vi "Mode_1.vi"(8 "error in (no error)":errorcluster, 11 "SetupInfo_IN":T1={"ConfigParameters_Analog"={"JAI camera fps"=240.0, "Bi-Lateral Galvo xy scan range (V)"=0.7, "Bi-Lateral Galvo xy scan frequency (Hz)"=500, "AOM Blind percent (%)"=0.1, "AOM start blind percent (%) "=70.0, "ROI threshold"=1.0, "AO Sampling rate"=1000000.0}, "ConfigParameters_Digital"={"Steps per volume"=25.0, "Time per volume (s)"=0.4, "OG start layer"=15.0, "Objective Lin Rising Vel (micron/ms）"=1.0, "Image depth (micron)"=200.0, "OG latency (s)"=10.0, "OG repitation"=3.0, "OG end layer"=17.0, "Shock1 duration (s)"=0.001, "Shock2 duration (s)"=0.001, "Shock3 duration (s)"=0.01, "Shock4 duration (s)"=0.01, "Shock5 duration (s)"=0.1, "Shock duration_New"=[]}, "ConfigParameters_Other1"={"Frontal Galvo xy scan range (V)"=0.14, "Frontal Galvo xy scan frequency (Hz)"=500, "PFI 0 digital clock frequency"=500000.0, "Window size for layer index"=0.5, "sCMOS fps"=95.0}, "ConfigParameters_Others2"={"#Trials baseline"=6, "#Trials test"=6, "Time before acq. (s)"=360.0, "Time before test (s)"=600.0, "#Blocks acquisition"=5, "Inter-trial interval baseline (s)"=60.0, "#Trials per acquition block"=6, "Inter-block interval acquisition (s)"=360.0, "Inter-trial interval acquisition (s)"=20.0, "Flash latency (s)"=10.0, "Flash duration (s)"=3.2, "Response duration (s)"=10.0, "MaxTimeEventDetection (s)"=6, "StimType"=enum."Flash", "#MaxEvents"=6}, "ProcessParametersOut"={"stand Z vol Acquisition time (s)"=0.2631578947368421, "stand Z vol Backward time (s)"=0.13684210526315793, "Objective scan volt"=5.0, "Bi-lateral Galvo Z scan volt"=0.1800000180000018, "Frontal Galvo Z scan volt"=0.14940000509752818, "Objective step length (micron)"=8.0, "OG Z volet Linear Dec time (s)"=0.024, "OG Z vol Stim. steps time (s)"=0.031578947368421054, "OG Z vol Linear Acc time (s)"=0.112, "#Vol. of flash"=8, "#Vol. of shock"=1, "#Vol. bef flash"=25, "#Vol. aft flash"=17, "OG Z vol Linear Dec time (s)"=0.112, "OG Z vol time (s)"=0.39073684210526316, "Stack duration"=[0.001, 0.001, 0.01, 0.01, 0.1], "AOM stand. value size"=400000, "Plane indexing length"=0, "#Vol. blank"=0, "#Vol. blank before acq"=0, "#Vol. blank before test"=0, " #Inter-block interval acquisition (Ed-St Vol)"=0}, "WaveformParameters"={"stand Z vol Acquisition samp info"={"Fs"=1000000.0, "#s"=263158.0}, "stand Z vol Backward samp info"={"Fs"=1000000.0, "#s"=136842.0}, "OG Z vol Linear Acc samp info"={"Fs"=1000000.0, "#s"=112000.0}, "OG Z vol Stim. steps samp info"={"Fs"=1000000.0, "#s"=31579.0}, "OG Z volet Linear Dec samp info"={"Fs"=1000000.0, "#s"=24000.0}, "OG Z vol Linear Dec samp info"={"Fs"=1000000.0, "#s"=112000.0}, "OG Z vol samp info"={"Fs"=1000000.0, "#s"=390737.0}, "stand Z vol backforth samp info"={"Fs"=1000000.0, "#s"=400000.0}}, "AnalogWaveform"={"Bi-lateral Galvo Z stand waveform"={"t0"=timestamp(0 s since 1904-01-01), "dt"=1.0, "Y"=[]}, "Frontal Galvo Z stand waveform"={"t0"=timestamp(0 s since 1904-01-01), "dt"=1.0, "Y"=[]}, "Bi-lateral Galvo XY stand waveform"={"t0"=timestamp(0 s since 1904-01-01), "dt"=1.0, "Y"=[]}, "Frontal Galvo XY stand waveform"={"t0"=timestamp(0 s since 1904-01-01), "dt"=1.0, "Y"=[]}, "sCMOS stand waveform"={"t0"=timestamp(0 s since 1904-01-01), "dt"=1.0, "Y"=[]}, "Detection objective stand waveform"={"t0"=timestamp(0 s since 1904-01-01), "dt"=1.0, "Y"=[]}, "AOM stand waveform"={"t0"=timestamp(0 s since 1904-01-01), "dt"=1.0, "Y"=[]}, "PFI 0 clock stand waveform"={"t0"=timestamp(0 s since 1904-01-01), "dt"=1.0, "Y"=[]}, "Bi-lateral Galvo Z OG waveform"={"t0"=timestamp(0 s since 1904-01-01), "dt"=1.0, "Y"=[]}, "Bi-lateral Galvo XY OG waveform"={"t0"=timestamp(0 s since 1904-01-01), "dt"=1.0, "Y"=[]}, "Frontal Galvo Z OG waveform"={"t0"=timestamp(0 s since 1904-01-01), "dt"=1.0, "Y"=[]}, "Frontal Galvo XY OG waveform"={"t0"=timestamp(0 s since 1904-01-01), "dt"=1.0, "Y"=[]}, "sCMOS OG waveform"={"t0"=timestamp(0 s since 1904-01-01), "dt"=1.0, "Y"=[]}, "Detection objective OG waveform"={"t0"=timestamp(0 s since 1904-01-01), "dt"=1.0, "Y"=[]}, "AOM OG waveform"={"t0"=timestamp(0 s since 1904-01-01), "dt"=1.0, "Y"=[]}, "PFI 0 clock OG wavee"={"t0"=timestamp(0 s since 1904-01-01), "dt"=1.0, "Y"=[]}, "sCMOS blank waveform"={"t0"=timestamp(0 s since 1904-01-01), "dt"=1.0, "Y"=[]}, "All analog OG wave"=[], "All analog stand wave"=[], "All analog blank wave"=[], "BufferWaveform_Analog"=[], "Bi-lateral Galvo Z XY"={"t0"=timestamp(0 s since 1904-01-01), "dt"=1.0, "Y"=[]}, "Frontal Galvo Z XY"={"t0"=timestamp(0 s since 1904-01-01), "dt"=1.0, "Y"=[]}, "sCMOS Trigger XY"={"t0"=timestamp(0 s since 1904-01-01), "dt"=1.0, "Y"=[]}, "Detection objective XY"={"t0"=timestamp(0 s since 1904-01-01), "dt"=1.0, "Y"=[]}, "AOM XY"={"t0"=timestamp(0 s since 1904-01-01), "dt"=1.0, "Y"=[]}, "Analog_XY"=[]}, "DigitalWaveform"={"AllDigitalStandWave"=[], "AllDigialEvokedWave"=[], "AllDigialOGWave"=[], "AllDigitalPairWave_1"=[], "AllDigitalPairWave_2"=[], "AllDigitalPairWave_3"=[], "AllDigitalPairWave_4"=[], "AllDigitalPairWave_5"=[], "Plane Indexing"={"t0"=timestamp(0 s since 1904-01-01), "dt"=0.0, "Y"={"transitions"=[], "data"=[]}, "error"={"status"=FALSE, "code"=37421928, "source"=""}}, "Plane indexing P0.5 OG"={"t0"=timestamp(0 s since 1904-01-01), "dt"=0.0, "Y"={"transitions"=[], "data"=[]}, "error"={"status"=FALSE, "code"=37421928, "source"=""}}, "AllDigitalPairWaves"=[], "BufferWaveform_Digital"=[], "AllDigitalBlankWave"=[], "Digial_XY"=[], "Digital_XY_flash"=[], "Digial_XY DMD"=[]}, "PhysicalResource"={"PhysicalChannels_AI"="", "PhysicalChannels_AO"="", "PhysicalChannels_DO"="", "Task_AnalogOutput"="", "Task_DigitalOutput"="", "Task_AnalogInput"=""}, "ControlsRef"={"Mode_1"=refnum, "EventDetectionMode"=refnum, "Mode_2A"=refnum, "StimulationMode"=refnum, "Mode_2B"=refnum, "ErrorMeg"=refnum}, "test"=""} {"ConfigParameters_Other1"."Frontal Galvo xy scan frequency (Hz)" min=500 max=500; "ConfigParameters_Other1"."Frontal Galvo xy scan range (V)" min=0.0 max=1.5; "ConfigParameters_Analog"."AOM start blind percent (%)" min=10.0 max=90.0; "ConfigParameters_Analog"."AOM Blind percent (%)" min=0.1 max=100.0; "ConfigParameters_Analog"."Bi-Lateral Galvo xy scan frequency (Hz)" min=500 max=500; "ConfigParameters_Analog"."Bi-Lateral Galvo xy scan range (V)" min=0.0 max=1.5}) -> (0 "error out":errorcluster, 3 "SetupInfo_OUT":T1={"ConfigParameters_Analog"={"JAI camera fps"=240.0, "Bi-Lateral Galvo xy scan range (V)"=0.7, "Bi-Lateral Galvo xy scan frequency (Hz)"=500, "AOM Blind percent (%)"=0.1, "AOM start blind percent (%) "=70.0, "ROI threshold"=1.0, "AO Sampling rate"=1000000.0}, "ConfigParameters_Digital"={"Steps per volume"=25.0, "Time per volume (s)"=0.4, "OG start layer"=15.0, "Objective Lin Rising Vel (micron/ms）"=1.0, "Image depth (micron)"=200.0, "OG latency (s)"=10.0, "OG repitation"=3.0, "OG end layer"=17.0, "Shock1 duration (s)"=0.001, "Shock2 duration (s)"=0.001, "Shock3 duration (s)"=0.01, "Shock4 duration (s)"=0.01, "Shock5 duration (s)"=0.1, "Shock duration_New"=[]}, "ConfigParameters_Other1"={"Frontal Galvo xy scan range (V)"=0.14, "Frontal Galvo xy scan frequency (Hz)"=500, "PFI 0 digital clock frequency"=500000.0, "Window size for layer index"=0.5, "sCMOS fps"=95.0}, "ConfigParameters_Others2"={"#Trials baseline"=6, "#Trials test"=6, "Time before acq. (s)"=360.0, "Time before test (s)"=600.0, "#Blocks acquisition"=5, "Inter-trial interval baseline (s)"=60.0, "#Trials per acquition block"=6, "Inter-block interval acquisition (s)"=360.0, "Inter-trial interval acquisition (s)"=20.0, "Flash latency (s)"=10.0, "Flash duration (s)"=3.2, "Response duration (s)"=10.0, "MaxTimeEventDetection (s)"=6, "StimType"=enum."Flash", "#MaxEvents"=6}, "ProcessParametersOut"={"stand Z vol Acquisition time (s)"=0.2631578947368421, "stand Z vol Backward time (s)"=0.13684210526315793, "Objective scan volt"=5.0, "Bi-lateral Galvo Z scan volt"=0.1800000180000018, "Frontal Galvo Z scan volt"=0.14940000509752818, "Objective step length (micron)"=8.0, "OG Z volet Linear Dec time (s)"=0.024, "OG Z vol Stim. steps time (s)"=0.031578947368421054, "OG Z vol Linear Acc time (s)"=0.112, "#Vol. of flash"=8, "#Vol. of shock"=1, "#Vol. bef flash"=25, "#Vol. aft flash"=17, "OG Z vol Linear Dec time (s)"=0.112, "OG Z vol time (s)"=0.39073684210526316, "Stack duration"=[0.001, 0.001, 0.01, 0.01, 0.1], "AOM stand. value size"=400000, "Plane indexing length"=0, "#Vol. blank"=0, "#Vol. blank before acq"=0, "#Vol. blank before test"=0, " #Inter-block interval acquisition (Ed-St Vol)"=0}, "WaveformParameters"={"stand Z vol Acquisition samp info"={"Fs"=1000000.0, "#s"=263158.0}, "stand Z vol Backward samp info"={"Fs"=1000000.0, "#s"=136842.0}, "OG Z vol Linear Acc samp info"={"Fs"=1000000.0, "#s"=112000.0}, "OG Z vol Stim. steps samp info"={"Fs"=1000000.0, "#s"=31579.0}, "OG Z volet Linear Dec samp info"={"Fs"=1000000.0, "#s"=24000.0}, "OG Z vol Linear Dec samp info"={"Fs"=1000000.0, "#s"=112000.0}, "OG Z vol samp info"={"Fs"=1000000.0, "#s"=390737.0}, "stand Z vol backforth samp info"={"Fs"=1000000.0, "#s"=400000.0}}, "AnalogWaveform"={"Bi-lateral Galvo Z stand waveform"={"t0"=timestamp(0 s since 1904-01-01), "dt"=1.0, "Y"=[]}, "Frontal Galvo Z stand waveform"={"t0"=timestamp(0 s since 1904-01-01), "dt"=1.0, "Y"=[]}, "Bi-lateral Galvo XY stand waveform"={"t0"=timestamp(0 s since 1904-01-01), "dt"=1.0, "Y"=[]}, "Frontal Galvo XY stand waveform"={"t0"=timestamp(0 s since 1904-01-01), "dt"=1.0, "Y"=[]}, "sCMOS stand waveform"={"t0"=timestamp(0 s since 1904-01-01), "dt"=1.0, "Y"=[]}, "Detection objective stand waveform"={"t0"=timestamp(0 s since 1904-01-01), "dt"=1.0, "Y"=[]}, "AOM stand waveform"={"t0"=timestamp(0 s since 1904-01-01), "dt"=1.0, "Y"=[]}, "PFI 0 clock stand waveform"={"t0"=timestamp(0 s since 1904-01-01), "dt"=1.0, "Y"=[]}, "Bi-lateral Galvo Z OG waveform"={"t0"=timestamp(0 s since 1904-01-01), "dt"=1.0, "Y"=[]}, "Bi-lateral Galvo XY OG waveform"={"t0"=timestamp(0 s since 1904-01-01), "dt"=1.0, "Y"=[]}, "Frontal Galvo Z OG waveform"={"t0"=timestamp(0 s since 1904-01-01), "dt"=1.0, "Y"=[]}, "Frontal Galvo XY OG waveform"={"t0"=timestamp(0 s since 1904-01-01), "dt"=1.0, "Y"=[]}, "sCMOS OG waveform"={"t0"=timestamp(0 s since 1904-01-01), "dt"=1.0, "Y"=[]}, "Detection objective OG waveform"={"t0"=timestamp(0 s since 1904-01-01), "dt"=1.0, "Y"=[]}, "AOM OG waveform"={"t0"=timestamp(0 s since 1904-01-01), "dt"=1.0, "Y"=[]}, "PFI 0 clock OG wavee"={"t0"=timestamp(0 s since 1904-01-01), "dt"=1.0, "Y"=[]}, "sCMOS blank waveform"={"t0"=timestamp(0 s since 1904-01-01), "dt"=1.0, "Y"=[]}, "All analog OG wave"=[], "All analog stand wave"=[], "All analog blank wave"=[], "BufferWaveform_Analog"=[], "Bi-lateral Galvo Z XY"={"t0"=timestamp(0 s since 1904-01-01), "dt"=1.0, "Y"=[]}, "Frontal Galvo Z XY"={"t0"=timestamp(0 s since 1904-01-01), "dt"=1.0, "Y"=[]}, "sCMOS Trigger XY"={"t0"=timestamp(0 s since 1904-01-01), "dt"=1.0, "Y"=[]}, "Detection objective XY"={"t0"=timestamp(0 s since 1904-01-01), "dt"=1.0, "Y"=[]}, "AOM XY"={"t0"=timestamp(0 s since 1904-01-01), "dt"=1.0, "Y"=[]}, "Analog_XY"=[]}, "DigitalWaveform"={"AllDigitalStandWave"=[], "AllDigialEvokedWave"=[], "AllDigialOGWave"=[], "AllDigitalPairWave_1"=[], "AllDigitalPairWave_2"=[], "AllDigitalPairWave_3"=[], "AllDigitalPairWave_4"=[], "AllDigitalPairWave_5"=[], "Plane Indexing"={"t0"=timestamp(0 s since 1904-01-01), "dt"=0.0, "Y"={"transitions"=[], "data"=[]}, "error"={"status"=FALSE, "code"=37421928, "source"=""}}, "Plane indexing P0.5 OG"={"t0"=timestamp(0 s since 1904-01-01), "dt"=0.0, "Y"={"transitions"=[], "data"=[]}, "error"={"status"=FALSE, "code"=37421928, "source"=""}}, "AllDigitalPairWaves"=[], "BufferWaveform_Digital"=[], "AllDigitalBlankWave"=[], "Digial_XY"=[], "Digital_XY_flash"=[], "Digial_XY DMD"=[]}, "PhysicalResource"={"PhysicalChannels_AI"="", "PhysicalChannels_AO"="", "PhysicalChannels_DO"="", "Task_AnalogOutput"="", "Task_DigitalOutput"="", "Task_AnalogInput"=""}, "ControlsRef"={"Mode_1"=refnum, "EventDetectionMode"=refnum, "Mode_2A"=refnum, "StimulationMode"=refnum, "Mode_2B"=refnum, "ErrorMeg"=refnum}, "test"=""} {"ConfigParameters_Other1"."Frontal Galvo xy scan frequency (Hz)" min=500 max=500; "ConfigParameters_Other1"."Frontal Galvo xy scan range (V)" min=0.0 max=1.5; "ConfigParameters_Analog"."AOM start blind percent (%)" min=10.0 max=90.0; "ConfigParameters_Analog"."AOM Blind percent (%)" min=0.1 max=100.0; "ConfigParameters_Analog"."Bi-Lateral Galvo xy scan frequency (Hz)" min=500 max=500; "ConfigParameters_Analog"."Bi-Lateral Galvo xy scan range (V)" min=0.0 max=1.5})   [LabVIEW 2018]
uses:
  SetupInfo.ctl
  ConfigParameters_Analog.ctl
  ConfigParameters_Digital.ctl
  ConfigParameters_Others1.ctl
  ConfigParameters_Others2.ctl
  ProcessParametersOut.ctl
  WaveformParameters.ctl
  AnalogWaveform.ctl
  DigitalWaveform.ctl
  PhysicalResource.ctl
  ControlsRef.ctl
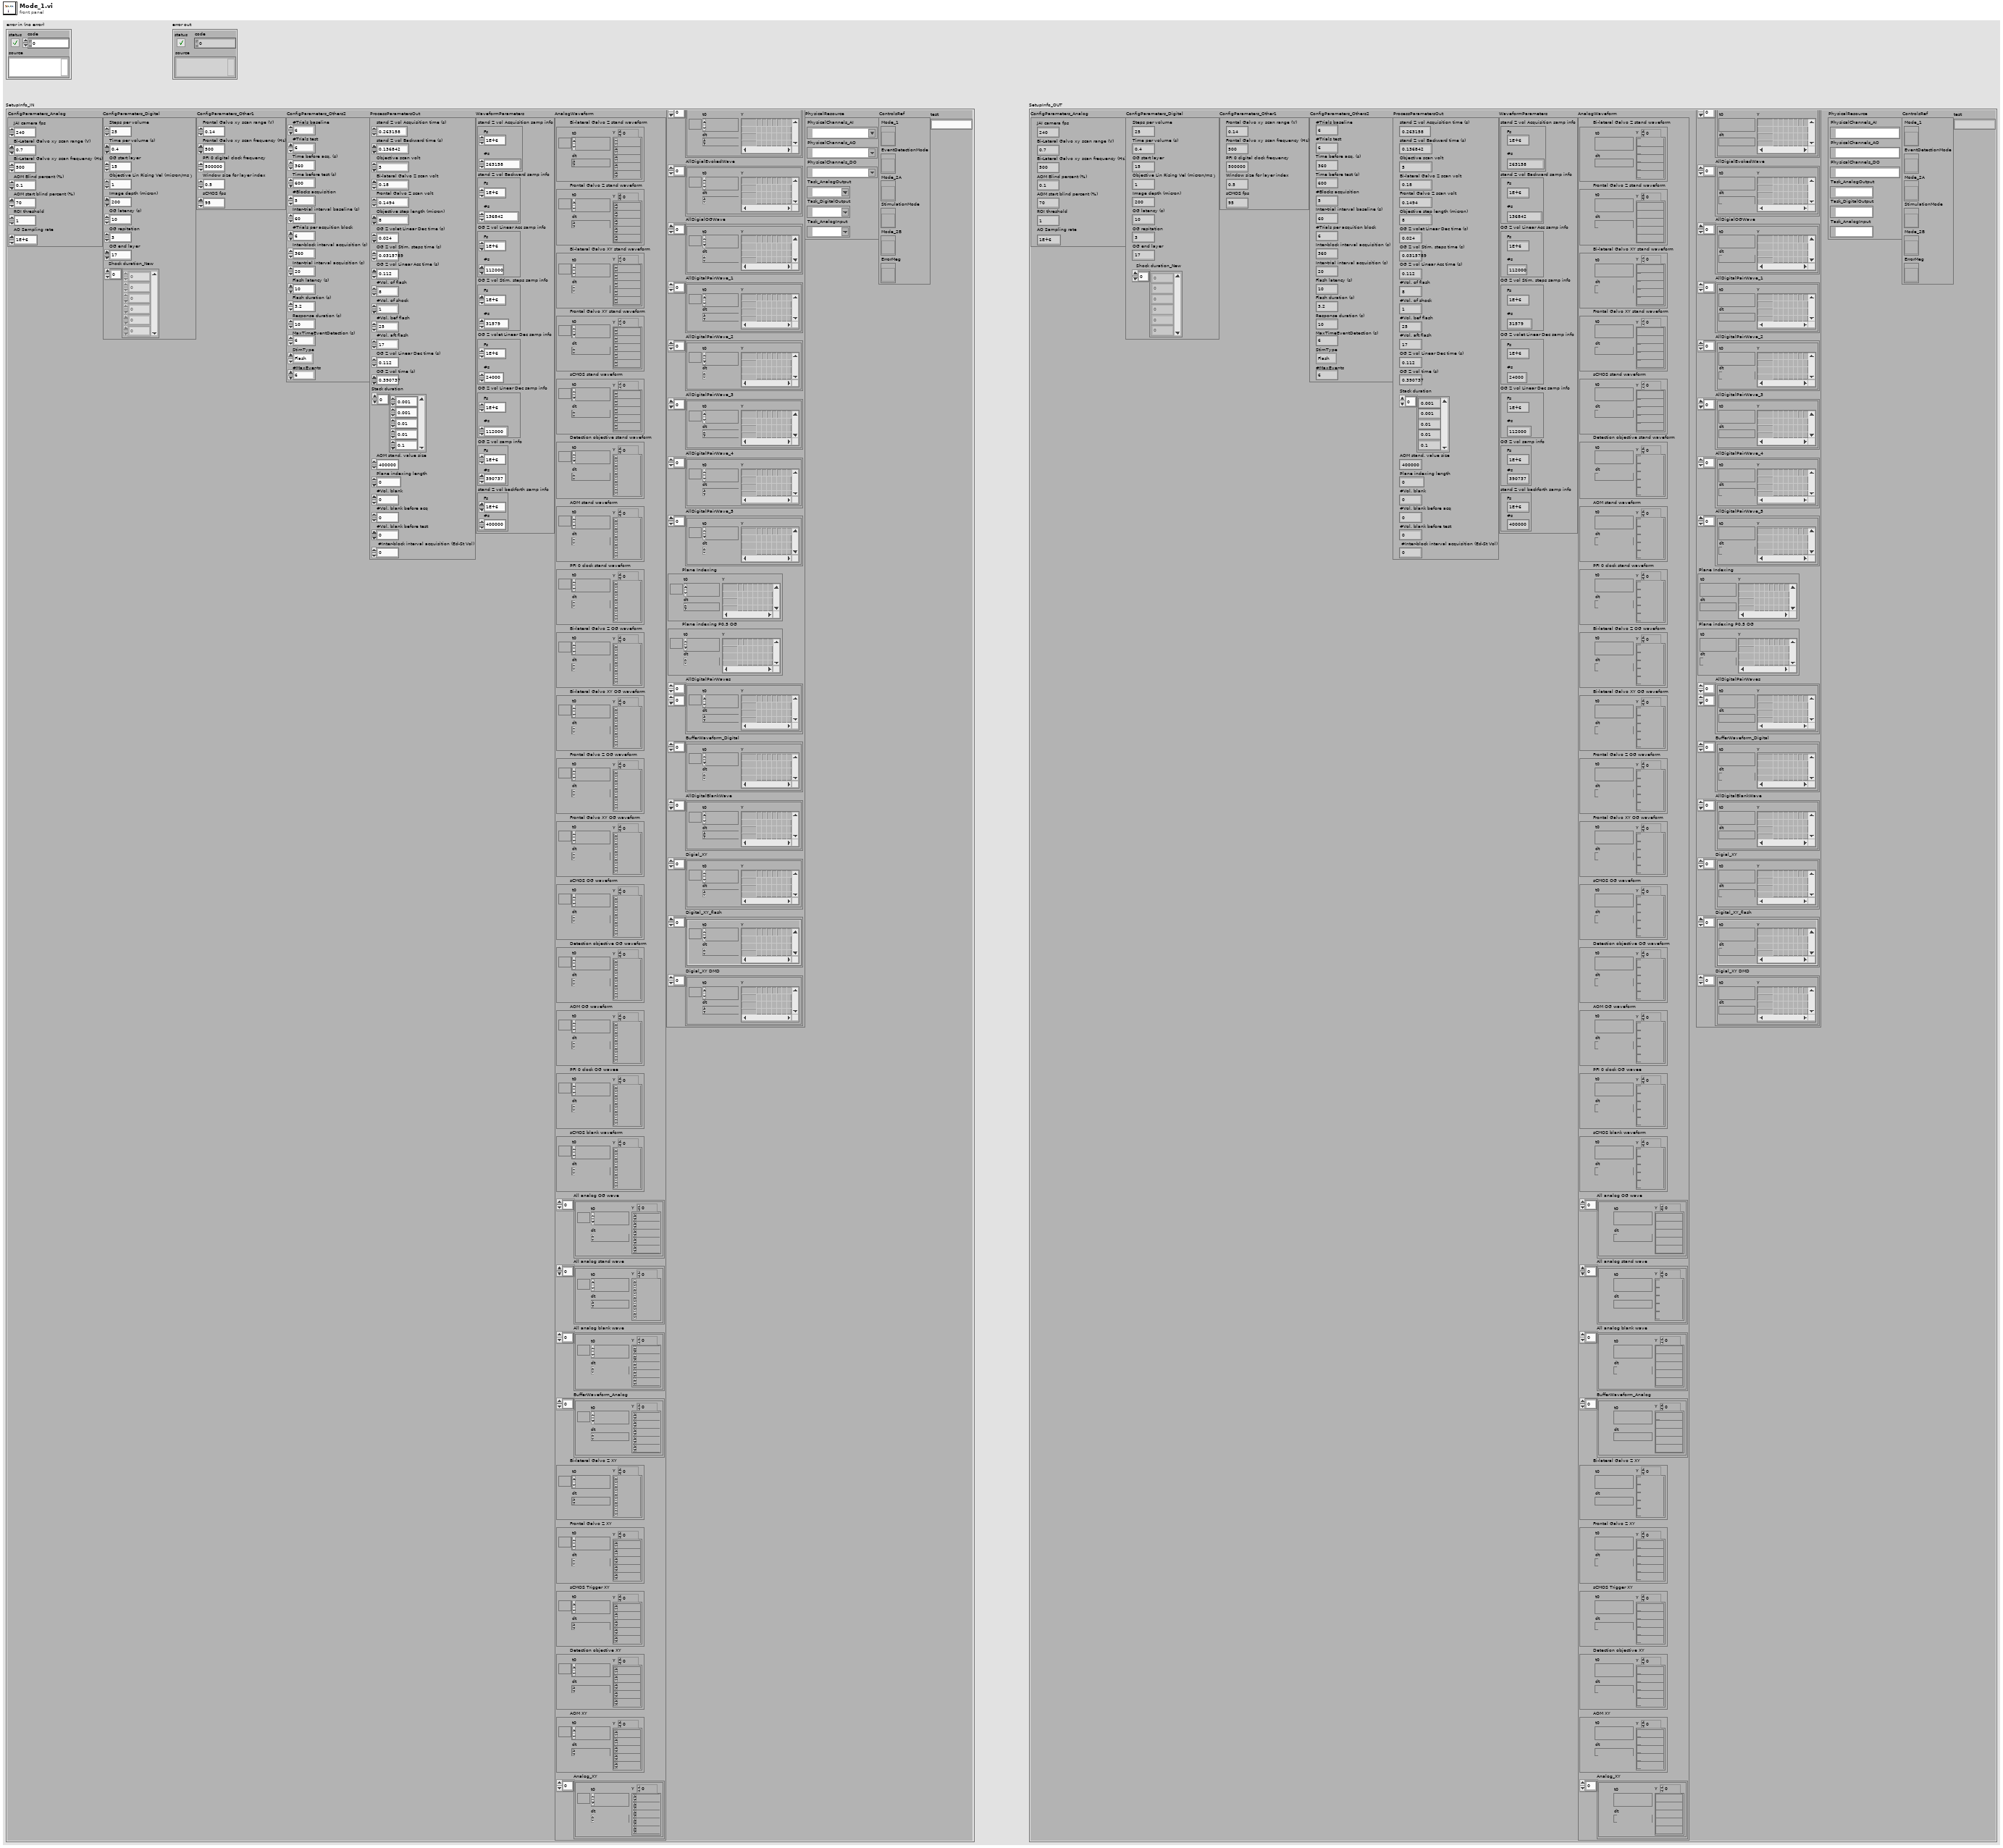
[diagram p1: front panel]
types:
  T1 = typedef "SetupInfo.ctl" = cluster{"ConfigParameters_Analog":T2, "ConfigParameters_Digital":T3, "ConfigParameters_Other1":T4, "ConfigParameters_Others2":T5, "ProcessParametersOut":T6, "WaveformParameters":T7, "AnalogWaveform":T8, "DigitalWaveform":T9, "PhysicalResource":T10, "ControlsRef":T11, "test":string}
  T2 = typedef "ConfigParameters_Analog.ctl" = cluster{"JAI camera fps":dbl, "Bi-Lateral Galvo xy scan range (V)":dbl, "Bi-Lateral Galvo xy scan frequency (Hz)":i16, "AOM Blind percent (%)":dbl, "AOM start blind percent (%) ":dbl, "ROI threshold":dbl, "AO Sampling rate":dbl}
  T3 = typedef "ConfigParameters_Digital.ctl" = cluster{"Steps per volume":dbl, "Time per volume (s)":dbl, "OG start layer":dbl, "Objective Lin Rising Vel (micron/ms）":dbl, "Image depth (micron)":dbl, "OG latency (s)":dbl, "OG repitation":dbl, "OG end layer":dbl, "Shock1 duration (s)":dbl, "Shock2 duration (s)":dbl, "Shock3 duration (s)":dbl, "Shock4 duration (s)":dbl, "Shock5 duration (s)":dbl, "Shock duration_New":dbl[]}
  T4 = typedef "ConfigParameters_Others1.ctl" = cluster{"Frontal Galvo xy scan range (V)":dbl, "Frontal Galvo xy scan frequency (Hz)":i16, "PFI 0 digital clock frequency":dbl, "Window size for layer index":dbl, "sCMOS fps":dbl}
  T5 = typedef "ConfigParameters_Others2.ctl" = cluster{"#Trials baseline":i32, "#Trials test":i32, "Time before acq. (s)":dbl, "Time before test (s)":dbl, "#Blocks acquisition":i32, "Inter-trial interval baseline (s)":dbl, "#Trials per acquition block":i32, "Inter-block interval acquisition (s)":dbl, "Inter-trial interval acquisition (s)":dbl, "Flash latency (s)":dbl, "Flash duration (s)":dbl, "Response duration (s)":dbl, "MaxTimeEventDetection (s)":i32, "StimType":enum16{"Flash", "OG"}, "#MaxEvents":i32}
  T6 = typedef "ProcessParametersOut.ctl" = cluster{"stand Z vol Acquisition time (s)":dbl, "stand Z vol Backward time (s)":dbl, "Objective scan volt":dbl, "Bi-lateral Galvo Z scan volt":dbl, "Frontal Galvo Z scan volt":dbl, "Objective step length (micron)":dbl, "OG Z volet Linear Dec time (s)":dbl, "OG Z vol Stim. steps time (s)":dbl, "OG Z vol Linear Acc time (s)":dbl, "#Vol. of flash":i32, "#Vol. of shock":i32, "#Vol. bef flash":i32, "#Vol. aft flash":i32, "OG Z vol Linear Dec time (s)":dbl, "OG Z vol time (s)":dbl, "Stack duration":dbl[], "AOM stand. value size":i32, "Plane indexing length":i32, "#Vol. blank":i32, "#Vol. blank before acq":i32, "#Vol. blank before test":i32, " #Inter-block interval acquisition (Ed-St Vol)":i32}
  T7 = typedef "WaveformParameters.ctl" = cluster{"stand Z vol Acquisition samp info":cluster{"Fs":dbl, "#s":dbl}, "stand Z vol Backward samp info":cluster{"Fs":dbl, "#s":dbl}, "OG Z vol Linear Acc samp info":cluster{"Fs":dbl, "#s":dbl}, "OG Z vol Stim. steps samp info":cluster{"Fs":dbl, "#s":dbl}, "OG Z volet Linear Dec samp info":cluster{"Fs":dbl, "#s":dbl}, "OG Z vol Linear Dec samp info":cluster{"Fs":dbl, "#s":dbl}, "OG Z vol samp info":cluster{"Fs":dbl, "#s":dbl}, "stand Z vol backforth samp info":cluster{"Fs":dbl, "#s":dbl}}
  T8 = typedef "AnalogWaveform.ctl" = cluster{"Bi-lateral Galvo Z stand waveform":waveform(dbl), "Frontal Galvo Z stand waveform":waveform(dbl), "Bi-lateral Galvo XY stand waveform":waveform(dbl), "Frontal Galvo XY stand waveform":waveform(dbl), "sCMOS stand waveform":waveform(dbl), "Detection objective stand waveform":waveform(dbl), "AOM stand waveform":waveform(dbl), "PFI 0 clock stand waveform":waveform(dbl), "Bi-lateral Galvo Z OG waveform":waveform(dbl), "Bi-lateral Galvo XY OG waveform":waveform(dbl), "Frontal Galvo Z OG waveform":waveform(dbl), "Frontal Galvo XY OG waveform":waveform(dbl), "sCMOS OG waveform":waveform(dbl), "Detection objective OG waveform":waveform(dbl), "AOM OG waveform":waveform(dbl), "PFI 0 clock OG wavee":waveform(dbl), "sCMOS blank waveform":waveform(dbl), "All analog OG wave":waveform(dbl)[], "All analog stand wave":waveform(dbl)[], "All analog blank wave":waveform(dbl)[], "BufferWaveform_Analog":waveform(dbl)[], "Bi-lateral Galvo Z XY":waveform(dbl), "Frontal Galvo Z XY":waveform(dbl), "sCMOS Trigger XY":waveform(dbl), "Detection objective XY":waveform(dbl), "AOM XY":waveform(dbl), "Analog_XY":waveform(dbl)[]}
  T9 = typedef "DigitalWaveform.ctl" = cluster{"AllDigitalStandWave":digitalwaveform[], "AllDigialEvokedWave":digitalwaveform[], "AllDigialOGWave":digitalwaveform[], "AllDigitalPairWave_1":digitalwaveform[], "AllDigitalPairWave_2":digitalwaveform[], "AllDigitalPairWave_3":digitalwaveform[], "AllDigitalPairWave_4":digitalwaveform[], "AllDigitalPairWave_5":digitalwaveform[], "Plane Indexing":digitalwaveform, "Plane indexing P0.5 OG":digitalwaveform, "AllDigitalPairWaves":digitalwaveform[][], "BufferWaveform_Digital":digitalwaveform[], "AllDigitalBlankWave":digitalwaveform[], "Digial_XY":digitalwaveform[], "Digital_XY_flash":digitalwaveform[], "Digial_XY DMD":digitalwaveform[]}
  T10 = typedef "PhysicalResource.ctl" = cluster{"PhysicalChannels_AI":tag, "PhysicalChannels_AO":tag, "PhysicalChannels_DO":tag, "Task_AnalogOutput":refnum<k21>, "Task_DigitalOutput":refnum<k21>, "Task_AnalogInput":refnum<k21>}
  T11 = typedef "ControlsRef.ctl" = cluster{"Mode_1":refnum<vi>, "EventDetectionMode":refnum<vi>, "Mode_2A":refnum<vi>, "StimulationMode":refnum<vi>, "Mode_2B":refnum<vi>, "ErrorMeg":refnum<vi>}
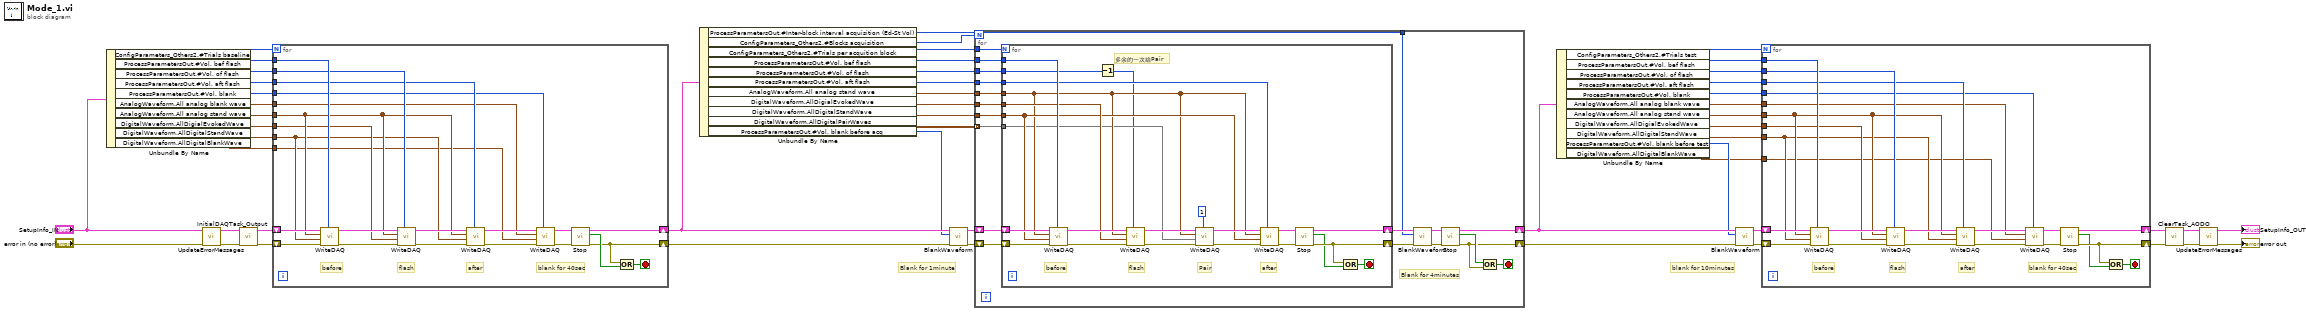
[diagram p0: block diagram]
diagram:
  # "blank for 10minutes"
  # "Blank for 1minute"
  n1 = Unbundle By Name("SetupInfo_IN") -> ("ConfigParameters_Others2.#Trials baseline"=w52:i32, "ProcessParametersOut.#Vol. bef flash"=w51:i32, "ProcessParametersOut.#Vol. of flash"=w50:i32, "ProcessParametersOut.#Vol. aft flash"=w49:i32, "ProcessParametersOut.#Vol. blank"=w48:i32, "AnalogWaveform.All analog blank wave"=w46:waveform(dbl)[], "AnalogWaveform.All analog stand wave"=w47:waveform(dbl)[], "DigitalWaveform.AllDigialEvokedWave"=w45:digitalwaveform[], "DigitalWaveform.AllDigitalStandWave"=w44:digitalwaveform[], "DigitalWaveform.AllDigitalBlankWave"=w2:digitalwaveform[])
  n2 = call "UpdateErrorMessages.vi"("error in (no error)"="error in (no error)", "SetupInfo_IN"="SetupInfo_IN") -> ("error out"=w4:errorcluster, "SetupInfo_OUT"=w3:T1)  [unwired: 8 in]
  n3 = call "InitialDAQTask_Output.vi"("error in (no error)"=w4, "SetupInfo_IN"=w3) -> ("error out"=w26:errorcluster, "SetupInfo_OUT"=w27:T1)  [unwired: 8 in]
  n4 = for {
    N: w52 -> [_]
    shift-right: [w54] -> w20
    shift-left: w26 -> [w72]
    tunnel: w51 -> [w70]
    shift-right: [w60] -> w21
    shift-left: w27 -> [w71]
    tunnel: w50 -> [w67]
    tunnel: w49 -> [w65]
    tunnel: w48 -> [w61]
    tunnel: w47 -> [w58]
    tunnel: w46 -> [w57]
    tunnel: w45 -> [w56]
    tunnel: w44 -> [w55]
    tunnel: w2 -> [w53]
    stop <- w73 stop-if-true
    # "blank for 40sec"
    # "after"
    # "flash"
    # "before"
    n5 = call "WriteDAQ.vi"("Cycle"=w70, "error in (no error)"=w72, "DigitalWaveform_In"=w55, "AnalogWaveform_In"=w58, "SetupInfo_IN"=w71) -> ("error out"=w69:errorcluster, "SetupInfo_OUT"=w68:T1)  [unwired: 4 in, 1 out]
    n6 = call "WriteDAQ.vi"("Cycle"=w67, "error in (no error)"=w69, "DigitalWaveform_In"=w56, "AnalogWaveform_In"=w58, "SetupInfo_IN"=w68) -> ("error out"=w66:errorcluster, "SetupInfo_OUT"=w64:T1)  [unwired: 4 in, 1 out]
    n7 = call "WriteDAQ.vi"("Cycle"=w65, "error in (no error)"=w66, "DigitalWaveform_In"=w55, "AnalogWaveform_In"=w58, "SetupInfo_IN"=w64) -> ("error out"=w63:errorcluster, "SetupInfo_OUT"=w62:T1)  [unwired: 4 in, 1 out]
    n8 = call "WriteDAQ.vi"("Cycle"=w61, "error in (no error)"=w63, "DigitalWaveform_In"=w53, "AnalogWaveform_In"=w57, "SetupInfo_IN"=w62) -> ("error out"=w59:errorcluster, "SetupInfo_OUT"=w60:T1)  [unwired: 4 in, 1 out]
    n9 = call "Stop.vi"("error in (no error)"=w59) -> ("error out"=w54:errorcluster, "StateOut"=w74:bool)  [unwired: 9 in]
    n10 = Compound Arithmetic op=OR(w54, w74) -> (w73:bool)
  }
  n11 = Unbundle By Name(w21) -> ("ProcessParametersOut.#Inter-block interval acquisition (Ed-St Vol)"=w11:i32, "ConfigParameters_Others2.#Blocks acquisition"=w22:i32, "ConfigParameters_Others2.#Trials per acquition block"=w37:i32, "ProcessParametersOut.#Vol. bef flash"=w38:i32, "ProcessParametersOut.#Vol. of flash"=w39:i32, "ProcessParametersOut.#Vol. aft flash"=w40:i32, "AnalogWaveform.All analog stand wave"=w41:waveform(dbl)[], "DigitalWaveform.AllDigialEvokedWave"=w42:digitalwaveform[], "DigitalWaveform.AllDigitalStandWave"=w43:digitalwaveform[], "DigitalWaveform.AllDigitalPairWaves"=w23:digitalwaveform[][], "ProcessParametersOut.#Vol. blank before acq"=w12:i32)
  n12 = call "BlankWaveform.vi"("error in (no error)"=w20, "Cycle"=w12, "SetupInfo_IN"=w21) -> ("error out"=w19:errorcluster, "SetupInfo_OUT"=w18:T1)  [unwired: 7 in]
  n13 = for {
    N: w22 -> [_]
    tunnel: w43 -> [w92]
    tunnel: w42 -> [w91]
    tunnel: w41 -> [w90]
    tunnel: w40 -> [w89]
    tunnel: w39 -> [w88]
    tunnel: w38 -> [w87]
    tunnel: w37 -> [w86]
    tunnel: w23 -> [w83] mode=indexing
    shift-right: [w77] -> w17
    shift-left: w18 -> [w85]
    shift-right: [w80] -> w14
    shift-left: w19 -> [w84]
    tunnel: w11 -> [w75]
    stop <- w81 stop-if-true
    # "Blank for 4minutes"
    n14 = for {
      N: w86 -> [_]
      shift-right: [w114] -> w79
      shift-left: w84 -> [w111]
      tunnel: w87 -> [w109]
      shift-right: [w100] -> w78
      shift-left: w85 -> [w110]
      tunnel: w88 -> [w106]
      tunnel: w89 -> [w101]
      tunnel: w90 -> [w96]
      tunnel: w91 -> [w98]
      tunnel: w92 -> [w97]
      tunnel: w83 -> [w95]
      stop <- w112 stop-if-true
      # "多余的一次给Pair"
      # "after"
      # "before"
      # "flash"
      # "Pair"
      n15 = call "WriteDAQ.vi"("Cycle"=w109, "error in (no error)"=w111, "DigitalWaveform_In"=w97, "AnalogWaveform_In"=w96, "SetupInfo_IN"=w110) -> ("error out"=w108:errorcluster, "SetupInfo_OUT"=w107:T1)  [unwired: 4 in, 1 out]
      n16 = Decrement(x=w106) -> (x-1=w93:i32)
      n17 = call "WriteDAQ.vi"("Cycle"=w93, "error in (no error)"=w108, "DigitalWaveform_In"=w98, "AnalogWaveform_In"=w96, "SetupInfo_IN"=w107) -> ("error out"=w105:errorcluster, "SetupInfo_OUT"=w104:T1)  [unwired: 4 in, 1 out]
      n18 = call "WriteDAQ.vi"("Cycle"=1, "error in (no error)"=w105, "DigitalWaveform_In"=w95, "AnalogWaveform_In"=w96, "SetupInfo_IN"=w104) -> ("error out"=w103:errorcluster, "SetupInfo_OUT"=w102:T1)  [unwired: 4 in, 1 out]
      n19 = call "WriteDAQ.vi"("Cycle"=w101, "error in (no error)"=w103, "DigitalWaveform_In"=w97, "AnalogWaveform_In"=w96, "SetupInfo_IN"=w102) -> ("error out"=w99:errorcluster, "SetupInfo_OUT"=w100:T1)  [unwired: 4 in, 1 out]
      n20 = call "Stop.vi"("error in (no error)"=w99) -> ("error out"=w114:errorcluster, "StateOut"=w113:bool)  [unwired: 9 in]
      n21 = Compound Arithmetic op=OR(w114, w113) -> (w112:bool)
    }
    n22 = call "BlankWaveform.vi"("error in (no error)"=w79, "Cycle"=w75, "SetupInfo_IN"=w78) -> ("error out"=w76:errorcluster, "SetupInfo_OUT"=w77:T1)  [unwired: 7 in]
    n23 = call "Stop.vi"("error in (no error)"=w76) -> ("error out"=w80:errorcluster, "StateOut"=w82:bool)  [unwired: 9 in]
    n24 = Compound Arithmetic op=OR(w82, w80) -> (w81:bool)
  }
  n25 = Unbundle By Name(w17) -> ("ConfigParameters_Others2.#Trials test"=w36:i32, "ProcessParametersOut.#Vol. bef flash"=w35:i32, "ProcessParametersOut.#Vol. of flash"=w34:i32, "ProcessParametersOut.#Vol. aft flash"=w33:i32, "ProcessParametersOut.#Vol. blank"=w32:i32, "AnalogWaveform.All analog blank wave"=w30:waveform(dbl)[], "AnalogWaveform.All analog stand wave"=w31:waveform(dbl)[], "DigitalWaveform.AllDigialEvokedWave"=w29:digitalwaveform[], "DigitalWaveform.AllDigitalStandWave"=w28:digitalwaveform[], "ProcessParametersOut.#Vol. blank before test"=w13:i32, "DigitalWaveform.AllDigitalBlankWave"=w1:digitalwaveform[])
  n26 = call "BlankWaveform.vi"("error in (no error)"=w14, "Cycle"=w13, "SetupInfo_IN"=w17) -> ("error out"=w15:errorcluster, "SetupInfo_OUT"=w16:T1)  [unwired: 7 in]
  n27 = for {
    N: w36 -> [_]
    shift-right: [w136] -> w24
    shift-left: w15 -> [w133]
    tunnel: w35 -> [w131]
    shift-right: [w121] -> w25
    shift-left: w16 -> [w132]
    tunnel: w34 -> [w128]
    tunnel: w33 -> [w126]
    tunnel: w32 -> [w122]
    tunnel: w31 -> [w119]
    tunnel: w30 -> [w118]
    tunnel: w29 -> [w117]
    tunnel: w28 -> [w116]
    tunnel: w1 -> [w115]
    stop <- w134 stop-if-true
    # "blank for 40sec"
    # "after"
    # "flash"
    # "before"
    n28 = call "WriteDAQ.vi"("Cycle"=w131, "error in (no error)"=w133, "DigitalWaveform_In"=w116, "AnalogWaveform_In"=w119, "SetupInfo_IN"=w132) -> ("error out"=w130:errorcluster, "SetupInfo_OUT"=w129:T1)  [unwired: 4 in, 1 out]
    n29 = call "WriteDAQ.vi"("Cycle"=w128, "error in (no error)"=w130, "DigitalWaveform_In"=w117, "AnalogWaveform_In"=w119, "SetupInfo_IN"=w129) -> ("error out"=w127:errorcluster, "SetupInfo_OUT"=w125:T1)  [unwired: 4 in, 1 out]
    n30 = call "WriteDAQ.vi"("Cycle"=w126, "error in (no error)"=w127, "DigitalWaveform_In"=w116, "AnalogWaveform_In"=w119, "SetupInfo_IN"=w125) -> ("error out"=w124:errorcluster, "SetupInfo_OUT"=w123:T1)  [unwired: 4 in, 1 out]
    n31 = call "WriteDAQ.vi"("Cycle"=w122, "error in (no error)"=w124, "DigitalWaveform_In"=w115, "AnalogWaveform_In"=w118, "SetupInfo_IN"=w123) -> ("error out"=w120:errorcluster, "SetupInfo_OUT"=w121:T1)  [unwired: 4 in, 1 out]
    n32 = call "Stop.vi"("error in (no error)"=w120) -> ("error out"=w136:errorcluster, "StateOut"=w135:bool)  [unwired: 9 in]
    n33 = Compound Arithmetic op=OR(w136, w135) -> (w134:bool)
  }
  n34 = call "ClearTask_AODO.vi"("error in (no error)"=w24, "SetupInfo_IN"=w25) -> ("error out"=w10:errorcluster, "SetupInfo_OUT"=w9:T1)  [unwired: 8 in]
  n35 = call "UpdateErrorMessages.vi"("error in (no error)"=w10, "SetupInfo_IN"=w9) -> ("error out"=→"error out":errorcluster, "SetupInfo_OUT"=→"SetupInfo_OUT":T1)  [unwired: 8 in]
